vi "Launcher.vi"() -> ()   [LabVIEW 2014, in "HIJ Vision App Fluence @ fix Energy Camera.lvlib"]
uses:
  HIJ Vision App Fluence @ fix Energy Camera.lvlib
  <vilib>/userdefined/High Color/IMAQdx.ctl
  HIJ Vision App Fluence and Energy Camera/HIJ Vision App Fluence @ fix Energy Camera.lvclass
  Applications/HIJ Vision Camera App/HIJ Vision Camera App/Write Start Camera.vi
  Applications/HIJ Vision Camera App/HIJ Vision Camera App/Write my ConfigDir.vi
  Applications/HIJ Vision Camera App/HIJ Vision Camera App/Write my WorkDir.vi
  Applications/HIJ Vision Camera App/HIJ Vision Camera App/Write Start Acquisition.vi
  <vilib>/ActorFramework/Actor/Actor.lvclass
panel:
  in  "Start WorkDir":path=path "C:/Users/user/Desktop/test/WorkDir"
  in  "Start ConfigDir":path=path "C:/Users/user/Desktop/test/ConfigDir"
  in  "Start Camera":T1="TestCam"
  out "error out":errorcluster
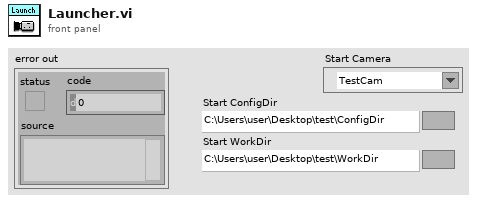
[diagram p1: front panel]
types:
  T1 = typedef "IMAQdx.ctl" = refnum<k21>
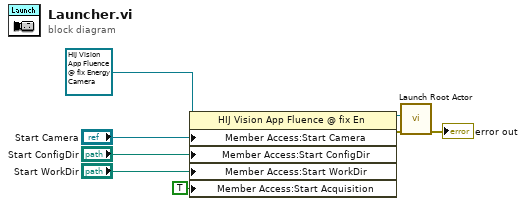
[diagram p0: block diagram]
diagram:
  n1 = property class="HIJ Vision App Fluence @ fix En"(reference=refnum<class "HIJ Vision App Fluence @ fix Energy Camera.lvclass"> refnum ("Launch IMAQ Display.lvlib:Launch IMAQ Display.lvclass"), "Member Access:Start Camera"="Start Camera", "Member Access:Start ConfigDir"="Start ConfigDir", "Member Access:Start WorkDir"="Start WorkDir", "Member Access:Start Acquisition"=TRUE ("Start Acquisition")) -> (reference out=w6:refnum<class "HIJ Vision App Fluence @ fix Energy Camera.lvclass">, error out=w5:errorcluster)  [unwired: 1 in]
  n2 = call <vilib>:"Launch Root Actor.vi"("error in (no error)"=w5, "Actor"=w6) -> ("error out"=→"error out":errorcluster)  [unwired: 8 in, 1 out]
